vi "Lissajou_Pattern.vi"() -> ()   [LabVIEW 2019]
uses:
  <vilib>/measure/NI_MABase.lvlib
panel:
  out "XY Graph":cluster{"Y":dbl[], "Y":dbl[]}[](graph)
  in  "B":dbl=1.0 format="%0.2p"
  in  "b":dbl=40.0 format="%0.2p"
  in  "sampling info":cluster{"Fs":dbl, "#s":dbl}={"Fs"=1000.0, "#s"=1000.0} {"Fs" format="%.2p"}
  in  "d":dbl=30.0 format="%.2p"
  in  "A":dbl=1.0 format="%0.2p"
  in  "a":dbl=50.0 format="%0.2p"
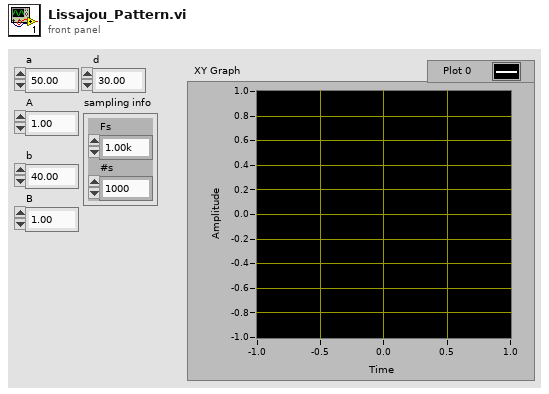
[diagram p1: front panel]
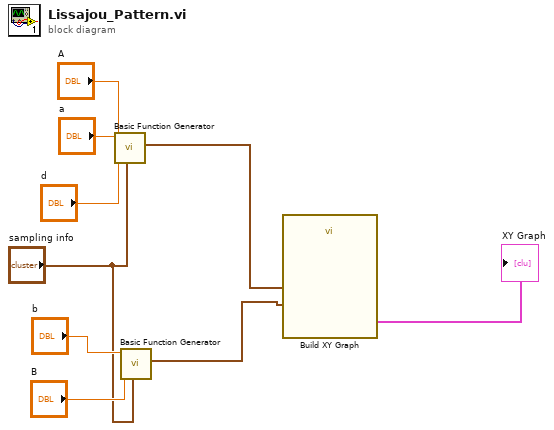
[diagram p0: block diagram]
diagram:
  n1 = call <vilib>:"Basic Function Generator.vi"("sampling info"="sampling info", "phase"="d", "amplitude"="A", "frequency"="a") -> ("signal out"=w2:waveform(dbl))  [unwired: 5 in, 2 out]
  n2 = call <vilib>:"Basic Function Generator.vi"("sampling info"="sampling info", "amplitude"="B", "frequency"="b") -> ("signal out"=w1:waveform(dbl))  [unwired: 6 in, 2 out]
  n3 = call "Build XY Graph"("Y Input"=w1, "X Input"=w2) -> ("XY Graph"=→"XY Graph":cluster{"X":dbl[], "Y":dbl[]}[])  [unwired: 8 in, 1 out]
